vi "Launch Viewer.vi"(6 "Subpanel ref lissajous":refnum<vi>, 7 "EMG?":bool=TRUE, 8 "error in (no error)":errorcluster, 9 "Collection Type":T1=enum."Movement Input", 10 "Subpanel ref task":refnum<vi>, 11 "NI Force Task in":refnum<class "NI Force Task.lvclass">) -> (0 "error out":errorcluster, 3 "NI Force Task out":refnum<class "NI Force Task.lvclass">)   [LabVIEW 2020, in "NI Force Task.lvlib" / "NI Force Task.lvclass"]
uses:
  NI Force Task.lvclass
  C:/Program Files/National Instruments/LabVIEW 2020/vi.lib/MGI/Panel Manager/Panel Actor/Panel Actor/Panel Actor.lvclass
  Collection Type df.ctl
  Task Viewer/Task Viewer.lvclass
  Lissajous Viewer/Lissajous Viewer.lvclass
  NI Force Task.lvclass/NI Force Task.ctl
  <vilib>/MGI/Panel Manager/Panel/Panel/Subpanel/Subpanel.lvclass
  C:/Program Files/National Instruments/LabVIEW 2020/vi.lib/MGI/Panel Manager/Panel/Panel/Panel.lvclass
  <vilib>/MGI/Panel Manager/Panel/Panel/Subpanel/Subpanel.vi
  <vilib>/MGI/Panel Manager/Panel Actor/Panel Actor/Panel Actor.lvclass
  <vilib>/MGI/Panel Manager/Panel/Panel.lvlib
  Task Viewer Messages/Set Legend Msg/Set Legend Msg.lvclass
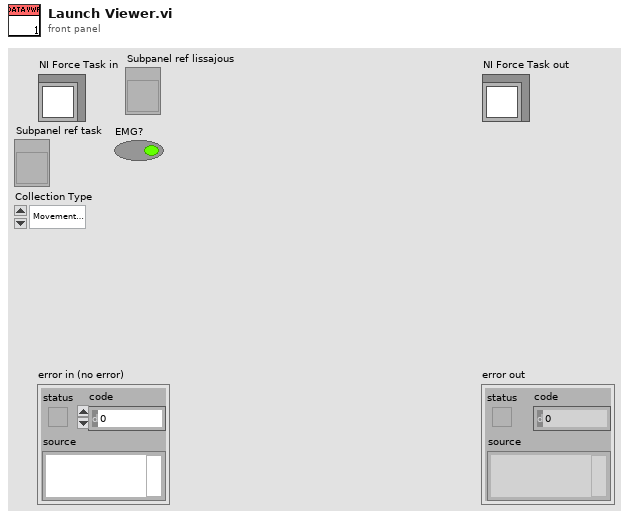
[diagram p1: front panel]
types:
  T1 = typedef "Collection Type df.ctl" = enum32{"Force Input", "Movement Input", "EMG only"}
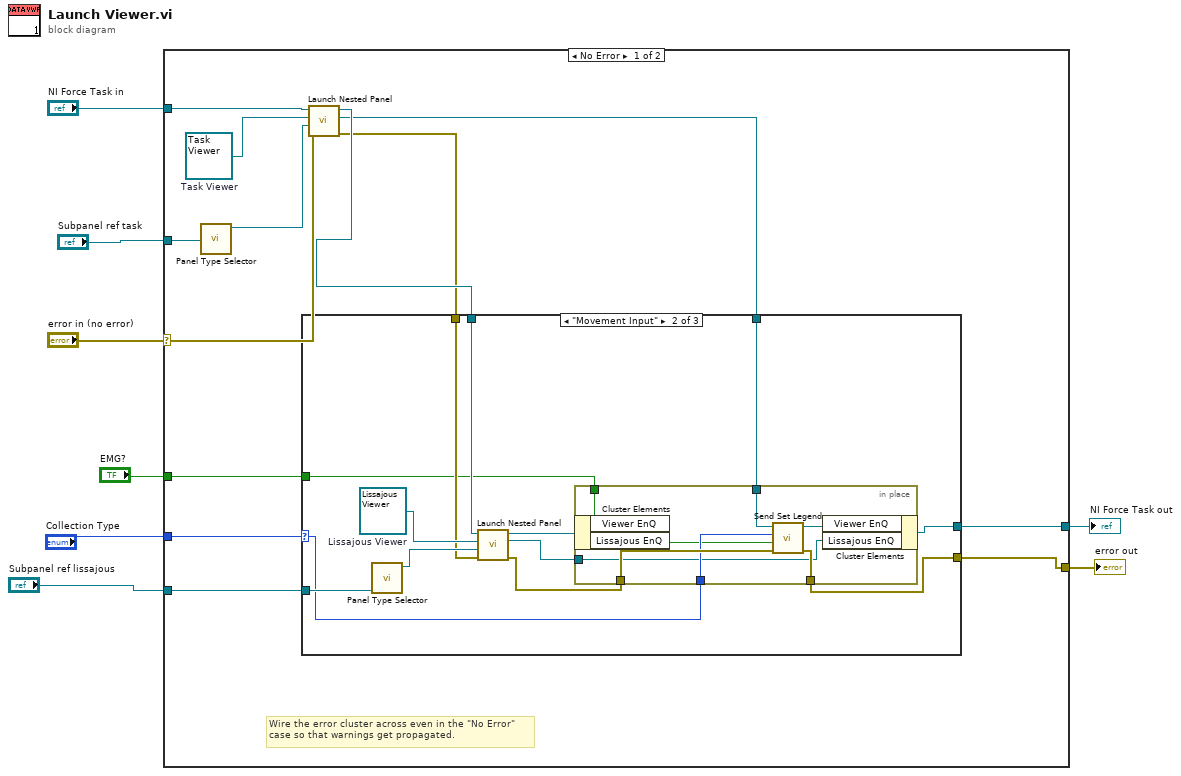
[diagram p0: block diagram]
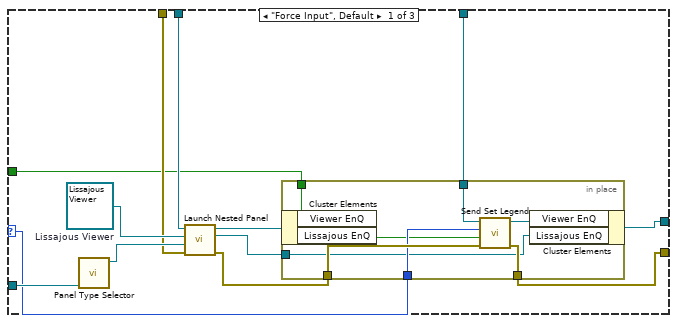
[diagram p2: hidden frame]
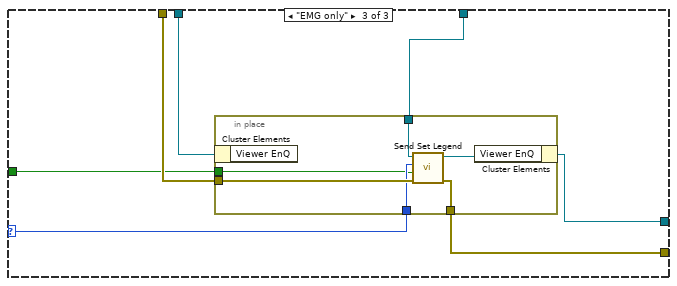
[diagram p3: hidden frame]
diagram:
  n1 = case shown="No Error" "error in (no error)" {
    selector: "error in (no error)" -> [w17 w76]
    tunnel: [w10 w76] -> w7
    tunnel: [w11 w75] -> w5
    tunnel: "NI Force Task in" -> [w21 w75]
    tunnel: "Subpanel ref task" -> [w18 _]
    tunnel: "Subpanel ref lissajous" -> [w15 _]
    tunnel: "Collection Type" -> [w13 _]
    tunnel: "EMG?" -> [w9 _]
    frame No Error {
      w20 = refnum<class "Task Viewer.lvclass"> refnum  # Task Viewer
      # "Wire the error cluster across even in the \"No Error\"\ncase so that warnings get propagated."
      n2 = call-poly <vilib>:"Panel Type Selector.vi"("Sub Panel"=w18) -> ("Subpanel Out"=w19:refnum<class "Subpanel.lvclass">)  [unwired: 9 in, 1 out]
      n3 = call <vilib>:"Launch Nested Panel.vi"("error in (no error)"=w17, "Panel"=w19, "Nested Panel Actor"=w20, "Panel Actor in"=w21) -> ("error out"=w14:errorcluster, "Nested Actor's Enqueuer"=w12:refnum<class "Message Enqueuer.lvclass">, "Panel Actor out"=w16:refnum<class "NI Force Task.lvclass">)  [unwired: 4 in, 1 out]
      n4 = case shown="\"Movement Input\"" w13 {
        selector: w13 -> [w27 w47 w63]
        tunnel: w16 -> [w33 w53 w68]
        tunnel: w15 -> [w31 w51 _]
        tunnel: w14 -> [w30 w50 w67]
        tunnel: [w23 w44 w66] -> w10
        tunnel: w12 -> [w26 w46 w64]
        tunnel: [w24 w43 w65] -> w11
        tunnel: w9 -> [w22 w42 w62]
        frame "Force Input", Default {
          w34 = refnum<class "Lissajous Viewer.lvclass"> refnum  # Lissajous Viewer
          n5 = call-poly <vilib>:"Panel Type Selector.vi"("Sub Panel"=w31) -> ("Subpanel Out"=w32:refnum<class "Subpanel.lvclass">)  [unwired: 9 in, 1 out]
          n6 = call <vilib>:"Launch Nested Panel.vi"("error in (no error)"=w30, "Panel"=w32, "Nested Panel Actor"=w34, "Panel Actor in"=w33) -> ("error out"=w28:errorcluster, "Nested Actor's Enqueuer"=w25:refnum<class "Message Enqueuer.lvclass">, "Panel Actor out"=w29:refnum<class "NI Force Task.lvclass">)  [unwired: 4 in, 1 out]
          n7 = in-place {
            in-place-border: [w40] -> w23
            in-place-border: w28 -> [w39]
            in-place-border: w27 -> [w38]
            in-place-border: w26 -> [w37]
            in-place-border: w25 -> [w36]
            in-place-border: w22 -> [w35]
            n8 = in-place-cluster #1(w29) -> ()  [unwired: 2 out]
            n9 = call "Send Set Legend.vi"("error in (no error)"=w39, "EMG?"=w35, "Collection mode"=w38, "Message Enqueuer in"=w37) -> ("error out"=w40:errorcluster, "Message Enqueuer out"=w41:refnum<class "Message Enqueuer.lvclass">)  [unwired: 6 in]
            n10 = in-place-cluster #1("Viewer EnQ"=w41, "Lissajous EnQ"=w36) -> (w24:refnum<class "NI Force Task.lvclass">)
          }
        }
        frame "Movement Input" {
          w54 = refnum<class "Lissajous Viewer.lvclass"> refnum  # Lissajous Viewer
          n11 = call-poly <vilib>:"Panel Type Selector.vi"("Sub Panel"=w51) -> ("Subpanel Out"=w52:refnum<class "Subpanel.lvclass">)  [unwired: 9 in, 1 out]
          n12 = call <vilib>:"Launch Nested Panel.vi"("error in (no error)"=w50, "Panel"=w52, "Nested Panel Actor"=w54, "Panel Actor in"=w53) -> ("error out"=w48:errorcluster, "Nested Actor's Enqueuer"=w45:refnum<class "Message Enqueuer.lvclass">, "Panel Actor out"=w49:refnum<class "NI Force Task.lvclass">)  [unwired: 4 in, 1 out]
          n13 = in-place {
            in-place-border: [w60] -> w44
            in-place-border: w48 -> [w59]
            in-place-border: w47 -> [w58]
            in-place-border: w46 -> [w57]
            in-place-border: w45 -> [w56]
            in-place-border: w42 -> [w55]
            n14 = in-place-cluster #2(w49) -> ()  [unwired: 2 out]
            n15 = call "Send Set Legend.vi"("error in (no error)"=w59, "EMG?"=w55, "Collection mode"=w58, "Message Enqueuer in"=w57) -> ("error out"=w60:errorcluster, "Message Enqueuer out"=w61:refnum<class "Message Enqueuer.lvclass">)  [unwired: 6 in]
            n16 = in-place-cluster #2("Viewer EnQ"=w61, "Lissajous EnQ"=w56) -> (w43:refnum<class "NI Force Task.lvclass">)
          }
        }
        frame "EMG only" {
          n17 = in-place {
            in-place-border: [w73] -> w66
            in-place-border: w67 -> [w72]
            in-place-border: w64 -> [w71]
            in-place-border: w63 -> [w70]
            in-place-border: w62 -> [w69]
            n18 = in-place-cluster #3(w68) -> ()  [unwired: 1 out]
            n19 = call "Send Set Legend.vi"("error in (no error)"=w72, "EMG?"=w69, "Collection mode"=w70, "Message Enqueuer in"=w71) -> ("error out"=w73:errorcluster, "Message Enqueuer out"=w74:refnum<class "Message Enqueuer.lvclass">)  [unwired: 6 in]
            n20 = in-place-cluster #3("Viewer EnQ"=w74) -> (w65:refnum<class "NI Force Task.lvclass">)
          }
        }
      }
    }
    frame Error {
    }
  }
  "error out" <- w7
  "NI Force Task out" <- w5
